vi "MSG display box two buttons.vi"(8 "error in":errorcluster, 9 "Enable":bool=TRUE, 10 "input string":string) -> (0 "error out":errorcluster, 1 "OK Button 2":bool)   [LabVIEW 2021]
panel:
  in  "Text.Text Colors:BG Color":u32(colorbox)=16448250
  out "String":string
  in  "OK Button":bool caption="Enter to OK"
  in  "Cancel":bool caption="ESC to Cancel"
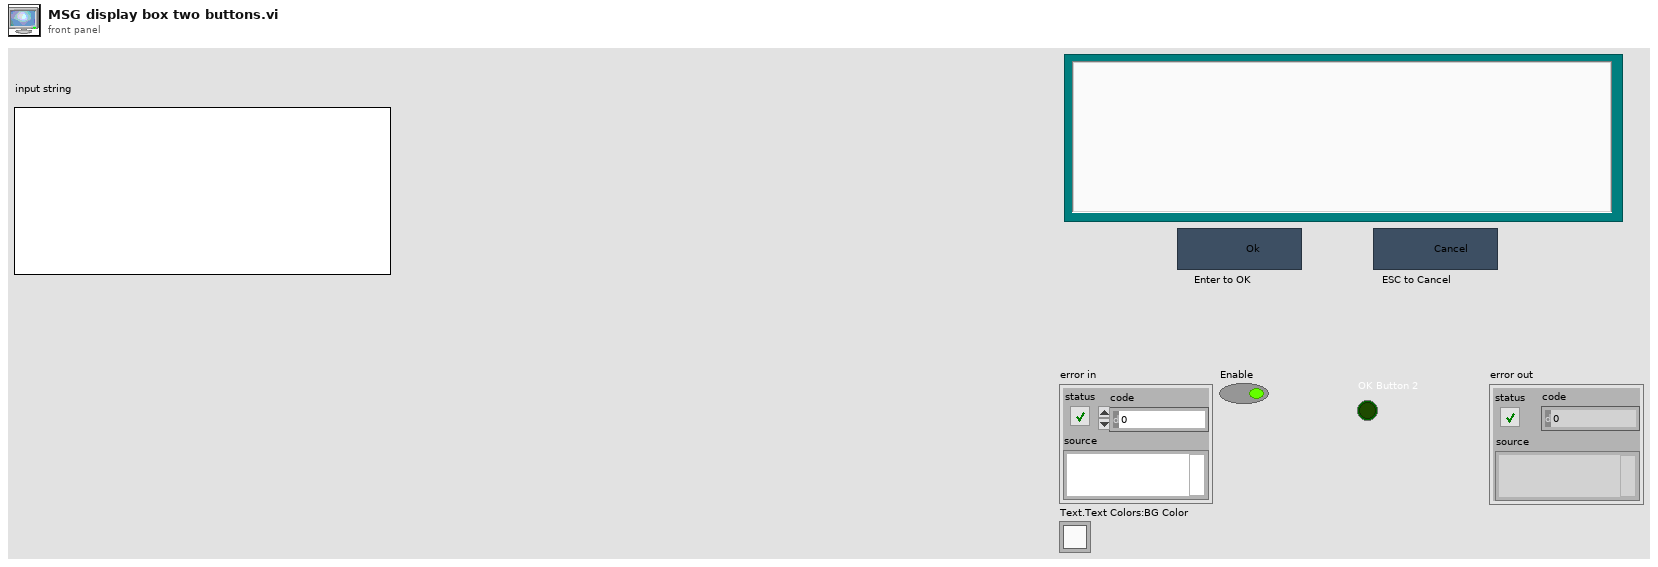
[diagram p1: front panel]
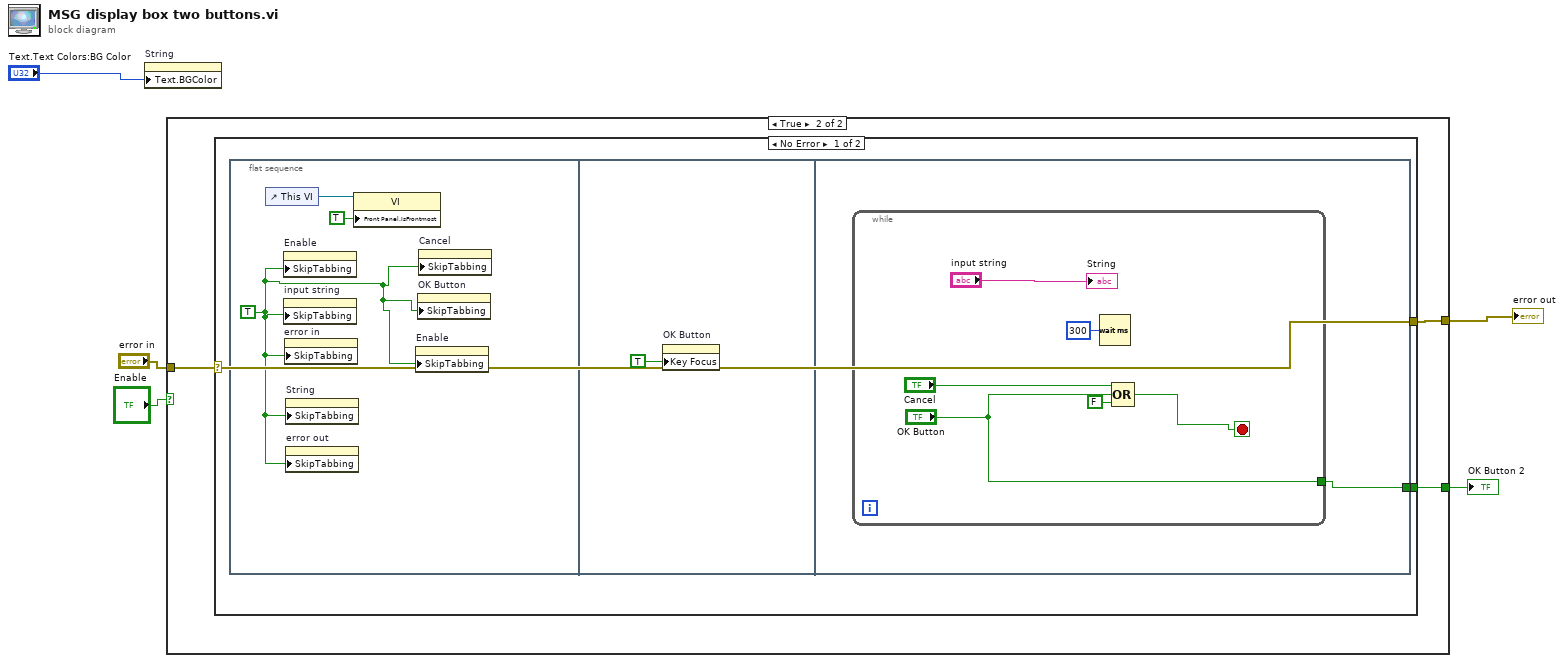
[diagram p0: block diagram]
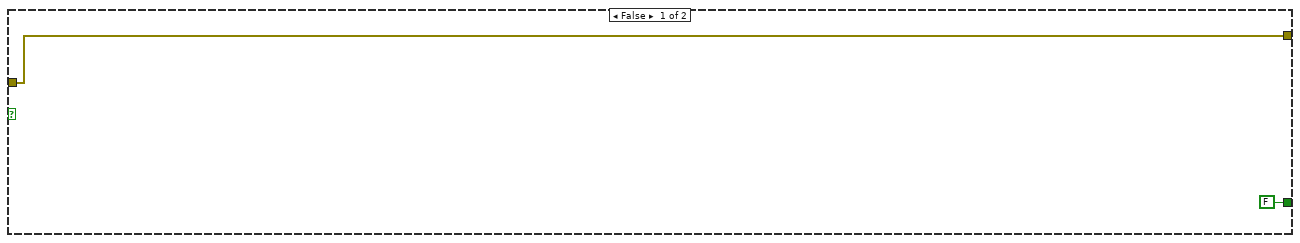
[diagram p2: hidden frame]
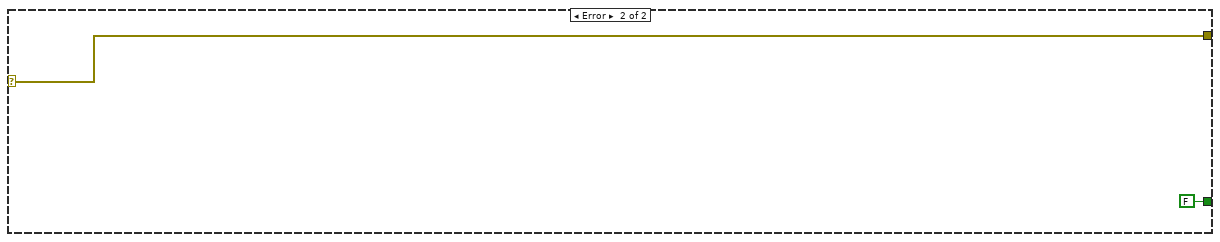
[diagram p3: hidden frame]
diagram:
  n1 = property on="String" class="Str"("Text.BGColor"="Text.Text Colors:BG Color") -> ()  [unwired: 2 in, 2 out]
  n2 = case shown="True" "Enable" {
    tunnel: "error in" -> [w7 w10]
    tunnel: [w7 w9] -> w4
    tunnel: [FALSE ("OK Button") w8] -> w1
    frame False {
    }
    frame True {
      n3 = case shown="No Error" w10 {
        selector: w10 -> [w12 w25]
        tunnel: [w12 w25] -> w9
        tunnel: [w11 FALSE ("OK Button")] -> w8
        frame No Error {
          n4 = flat-sequence {
            tunnel: [w17] -> w11
            frame #0 {
              w13 = TRUE ("Skip When Tabbing")
              n5 = control-ref of="This VI"() -> (w15:refnum<vi>)
              n6 = property on="Enable" class="Bool (strict)"("SkipTabbing"=w13) -> ()  [unwired: 2 in, 2 out]
              n7 = property on="input string" class="Str"("SkipTabbing"=w13) -> ()  [unwired: 2 in, 2 out]
              n8 = property on="error in" class="Clust (strict)"("SkipTabbing"=w13) -> ()  [unwired: 2 in, 2 out]
              n9 = property on="String" class="Str"("SkipTabbing"=w13) -> ()  [unwired: 2 in, 2 out]
              n10 = property on="error out" class="Clust (strict)"("SkipTabbing"=w13) -> ()  [unwired: 2 in, 2 out]
              n11 = property class="VI"(reference=w15, "Front Panel.IsFrontmost"=TRUE ("Front Panel Window:Is Frontmost")) -> ()  [unwired: 1 in, 2 out]
              n12 = property on="Enable" class="Bool (strict)"("SkipTabbing"=w13) -> ()  [unwired: 2 in, 2 out]
              n13 = property on="OK Button" class="Bool"("SkipTabbing"=w13) -> ()  [unwired: 2 in, 2 out]
              n14 = property on="Cancel" class="Bool"("SkipTabbing"=w13) -> ()  [unwired: 2 in, 2 out]
            }
            frame #1 {
              n15 = property on="OK Button" class="Bool"("Key Focus"=TRUE) -> ()  [unwired: 2 in, 2 out]
            }
            frame #2 {
              n16 = while {
                tunnel: ["OK Button"] -> w17
                stop <- w19 stop-if-true
                n17 = Wait (ms)(milliseconds to wait=u32 300) -> ()  [unwired: 1 out]
                n18 = Compound Arithmetic op=OR("Cancel", "OK Button", FALSE ("value")) -> (w19:bool)
                "String" <- "input string"
              }
            }
          }
        }
        frame Error {
        }
      }
    }
  }
  "error out" <- w4
  "OK Button 2" <- w1
